vi "Automatically Configure Gyro Offset.vi"(8 "error in (no error)":errorcluster, 9 "Sample Time (10000 ms)":u16=10000, 11 "VISA resource name":refnum<visa-resource-name>) -> (0 "error out":errorcluster, 3 "VISA resource name out":refnum<visa-resource-name>)   [LabVIEW 2012, in "MicroStrain 3DM-GXx.lvlib"]
doc: "Have the device sample its sensors for the specified time (ms) and determine the average gyro offset. This offset will automatically be written to the device's GyroBias vector and subtracted from subsequent Angular Rate measurements.\n\nRecommended sample times are 10,000 to 30,000 ms.\n\nThe device must be stationary for the duration of the sample time.\n\nThe offset vector is stored in the device's RAM and will be lost when the device loses power."
uses:
  <instrlib>/MicroStrain 3DM-GXx/MicroStrain 3DM-GXx.lvlib
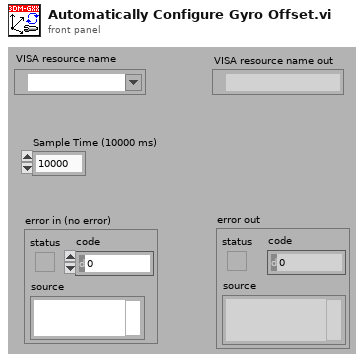
[diagram p1: front panel]
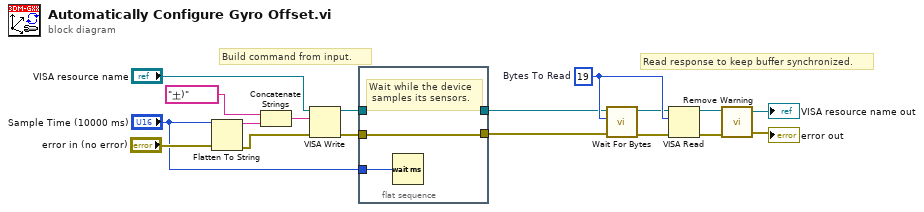
[diagram p0: block diagram]
diagram:
  w10 = u32 19  # Bytes To Read
  # "Read response to keep buffer synchronized."
  # "Build command from input."
  n1 = Flatten To String(anything="Sample Time (10000 ms)", error in (no error)="error in (no error)") -> (data string=w12:string, error out=w5:errorcluster)  [unwired: 2 in, 1 out]
  n2 = Concatenate Strings("土)", w12) -> (w13:string)
  n3 = VISA Write(VISA resource name="VISA resource name", write buffer=w13, error in (no error)=w5) -> (VISA resource name out=w1:refnum<visa-resource-name>, error out=w3:errorcluster)  [unwired: 1 out]
  n4 = flat-sequence {
    tunnel: "Sample Time (10000 ms)" -> [w21]
    tunnel: [w20] -> w4
    tunnel: w3 -> [w20]
    tunnel: [w19] -> w2
    tunnel: w1 -> [w19]
    frame #0 {
      # "Wait while the device\n samples its sensors."
      n5 = Wait (ms)(milliseconds to wait=w21) -> ()  [unwired: 1 out]
    }
  }
  n6 = call <instrlib>:"Wait For Bytes.vi"("error in (no error)"=w4, "Bytes To Read (0)"=w10, "VISA resource name"=w2) -> ("error out"=w9:errorcluster, "VISA resource name out"=w8:refnum<visa-resource-name>)  [unwired: 7 in]
  n7 = VISA Read(VISA resource name=w8, byte count=w10, error in (no error)=w9) -> (VISA resource name out=w7:refnum<visa-resource-name>, error out=w6:errorcluster)  [unwired: 2 out]
  n8 = call <instrlib>:"Remove Warning.vi"("error in (no error)"=w6, "VISA resource name"=w7) -> ("error out"=→"error out":errorcluster, "VISA resource name out"=→"VISA resource name out":refnum<visa-resource-name>)  [unwired: 2 in]
